vi "balance_controller.vi"(8 "Other variables":T1, 9 "systems":T6 {"SysD"."Transport Delay" format="%.2f"; "SysD"."D" format="%#.2g"; "SysD"."C" format="%#.2g"; "SysD"."B" format="%#.2g"; "SysD"."A" format="%#.2g"; "SysD"."properties"."Sampling Time" format="%#.6p"; "SysD"."properties"."Output Delays" format="%.4f"; "SysD"."properties"."Input Delays" format="%.4f"; "sysDo"."Transport Delay" format="%.2f"; "sysDo"."D" format="%#.2g"; "sysDo"."C" format="%#.2g"; "sysDo"."B" format="%#.2g"; "sysDo"."A" format="%#.2g"; "sysDo"."properties"."Sampling Time" format="%#.6p"; "sysDo"."properties"."Output Delays" format="%.4f"; "sysDo"."properties"."Input Delays" format="%.4f"; "sysDi"."Transport Delay" format="%.2f"; "sysDi"."D" format="%#.2g"; "sysDi"."C" format="%#.2g"; "sysDi"."B" format="%#.2g"; "sysDi"."A" format="%#.2g"; "sysDi"."properties"."Sampling Time" format="%#.6p"; "sysDi"."properties"."Output Delays" format="%.4f"; "sysDi"."properties"."Input Delays" format="%.4f"; "sysDC"."transfer function(s)"."delay" format="%.4f"; "sysDC"."transfer function(s)"."Denominator" format="%#_3g"; "sysDC"."transfer function(s)"."Numerator" format="%#_3g"; "sysDC"."properties"."Sampling Time" format="%#.6p"; "sysDC"."properties"."Output Delays" format="%.4f"; "sysDC"."properties"."Input Delays" format="%.4f"}) -> (3 "motor direction":dbl)   [LabVIEW 2016]
uses:
  <vilib>/addons/Control Design/_Model Construction/Model Typedefs.llb/CD State Space Model (MIMO).ctl
  <vilib>/addons/Control Design/_Model Construction/Model Typedefs.llb/CD General Elements.ctl
  <vilib>/addons/Control Design/_Model Construction/Model Typedefs.llb/CD Transfer Function Model (MIMO).ctl
  <vilib>/addons/Control Design/_Model Construction/Model Typedefs.llb/CD Transfer Function Model (SISO).ctl
  <vilib>/Analysis/Matrix/Datatypes/RealMatrix.ctl
  <vilib>/Simulation/DiscreteLinear/Implementation/NILVSim Discrete Transfer Function Direct.llb/SIM Discrete Transfer Function Diagram (SISO).vi
  <vilib>/Analysis/baseanly.llb/Real A x B.vi
  <vilib>/Simulation/ContinuousLinear/Implementation/Shared/SIM Transfer Function Support.llb/SIM TransferFunction Normalize to Buffer.vi
  <vilib>/Simulation/DiscreteLinear/Implementation/Shared/SIM Init Discrete States.vi
  <vilib>/Simulation/DiscreteLinear/Implementation/NILVSim Discrete Transfer Function Direct.llb/SIM Transfer Function Direct core (SISO).vi
  <vilib>/Simulation/ContinuousLinear/Implementation/Shared/SIM Transfer Function Support.llb/SIM TransferFunction Normalize.vi
  <vilib>/Simulation/Implementation/Shared/SIM Polynomials.llb/SIM Remove Zero Coefficients (DBL).vi
  <vilib>/Simulation/Implementation/Shared/SIM Polynomials.llb/SIM Divide Polynomials (DBL).vi
  <vilib>/Simulation/Implementation/Shared/SIM BuildSimErr.vi
  <vilib>/Analysis/Matrix/Numeric/Subtract/Subtract (Elementwise) - R,RM.vi
  <vilib>/Analysis/Matrix/Numeric/Add/Add - RM,RM.vi
  <vilib>/Simulation/Implementation/XNodeFramework/SimXNode/SimX.xnode
  <vilib>/Analysis/NI_AALBase.lvlib
  <vilib>/Simulation/ContinuousLinear/Implementation/NILVSim Integrator new.llb/SIM Integrator (vector).vi
  <vilib>/Analysis/baseanly.llb/A x Vector.vi
  <vilib>/Simulation/ContinuousLinear/Implementation/NILVSim Transfer Function.llb/SIM Transfer Function (SISO).vi
  <vilib>/Simulation/Nonlinear/Implementation/NILVSim Saturation.llb/SIM Saturation (scalar).vi
  <vilib>/Simulation/SignalDisplay/Implementation/NILVSim Time Waveform.llb/SIM Time Waveform (vector).vi
  <vilib>/Simulation/Nonlinear/Implementation/NILVSim Saturation.llb/SIM Saturation (vector).vi
  <vilib>/Analysis/baseanly.llb/Dot Product.vi
  <vilib>/Analysis/baseanly.llb/Real Dot Product.vi
  <vilib>/Simulation/Scripting/Companion Diagram/SimConfigNode/SimDog.xnode
  <vilib>/Simulation/Scripting/Companion Diagram/SimConfigNode/SimParams.ctl
  <vilib>/Simulation/Implementation/Shared/SIMSCR Execution Mode.ctl
  <vilib>/Simulation/Scripting/Companion Diagram/SimConfigNode/_simSolvers.ctl
  <vilib>/Simulation/Implementation/Shared/SIM Bundle Sim Info.vi
  <vilib>/Simulation/Implementation/Shared/SIM Unbundle Sim Info.vi
  <vilib>/Simulation/Implementation/Shared/NILVSim_FinalizeModel.vi
  <vilib>/Simulation/Implementation/Shared/NILVSim_GetModelError.vi
  <vilib>/Simulation/Implementation/Shared/NILVSim_Initialize.vi
  <vilib>/Simulation/Utility/Implementation/NILVSim Get Time and IsAcceptedStep.vi
  <vilib>/Simulation/Implementation/Shared/NILVSim_Manager.vi
  <vilib>/Simulation/Implementation/Shared/NI_SIM_Implementation.lvlib
  <vilib>/Simulation/Implementation/Shared/NILVSIM_BeginStep.vi
  <vilib>/Simulation/Param Hierarchy/Typedefs/SIMPH Param Control Actions.ctl
  <vilib>/Simulation/Implementation/Shared/NILVSim_ParamChanged.vi
  <vilib>/Utility/error.llb/Clear Errors.vi
  <vilib>/Simulation/Implementation/Shared/SIMSH Read Queue.vi
  <vilib>/Simulation/ContinuousLinear/Implementation/NILVSim Integrator new.llb/SIM Integrator Collector (vector).vi
  <vilib>/Simulation/ContinuousLinear/Implementation/NILVSim Integrator new.llb/SIM Integrator Distributor (vector).vi
  <vilib>/Simulation/Implementation/Shared/SIM limit type.ctl
  <vilib>/Simulation/ContinuousLinear/Implementation/NILVSim Transfer Function.llb/SIM Transfer Function Collector (SISO).vi
  <vilib>/Simulation/ContinuousLinear/Implementation/NILVSim Transfer Function.llb/SIM Transfer Function Distributor (SISO).vi
  <vilib>/Analysis/Matrix/NI_Matrix.lvlib
  <vilib>/Simulation/DiscreteLinear/Implementation/NILVSim Discrete Transfer Function Buffered.llb/SIM Discrete Transfer Function Buffered (SISO).vi
  <vilib>/Simulation/DiscreteLinear/Implementation/NILVSim Discrete Transfer Function Buffered.llb/SIM Discrete Transfer Function Distributor (SISO).vi
  <vilib>/addons/Control Design/_Model Construction/NI_LinSys_Model Typedefs.lvlib
panel:
  out "Waveform Chart 5":dbl[](graph)
  out "Waveform Chart 4":dbl[](graph)
  out "Waveform Chart 3":dbl[](graph)
  out "Waveform Chart 2":dbl[](graph)
  out "Waveform Chart":waveform(dbl)[](graph)
  in  "Whipple":T7
  out "Error":errorcluster
  out "output cluster":cluster{dbl[], dbl[]}
  in  "Inner Control Variable":T8
  in  "Outer Control Variable":T9
  in  "Other Variables":T10
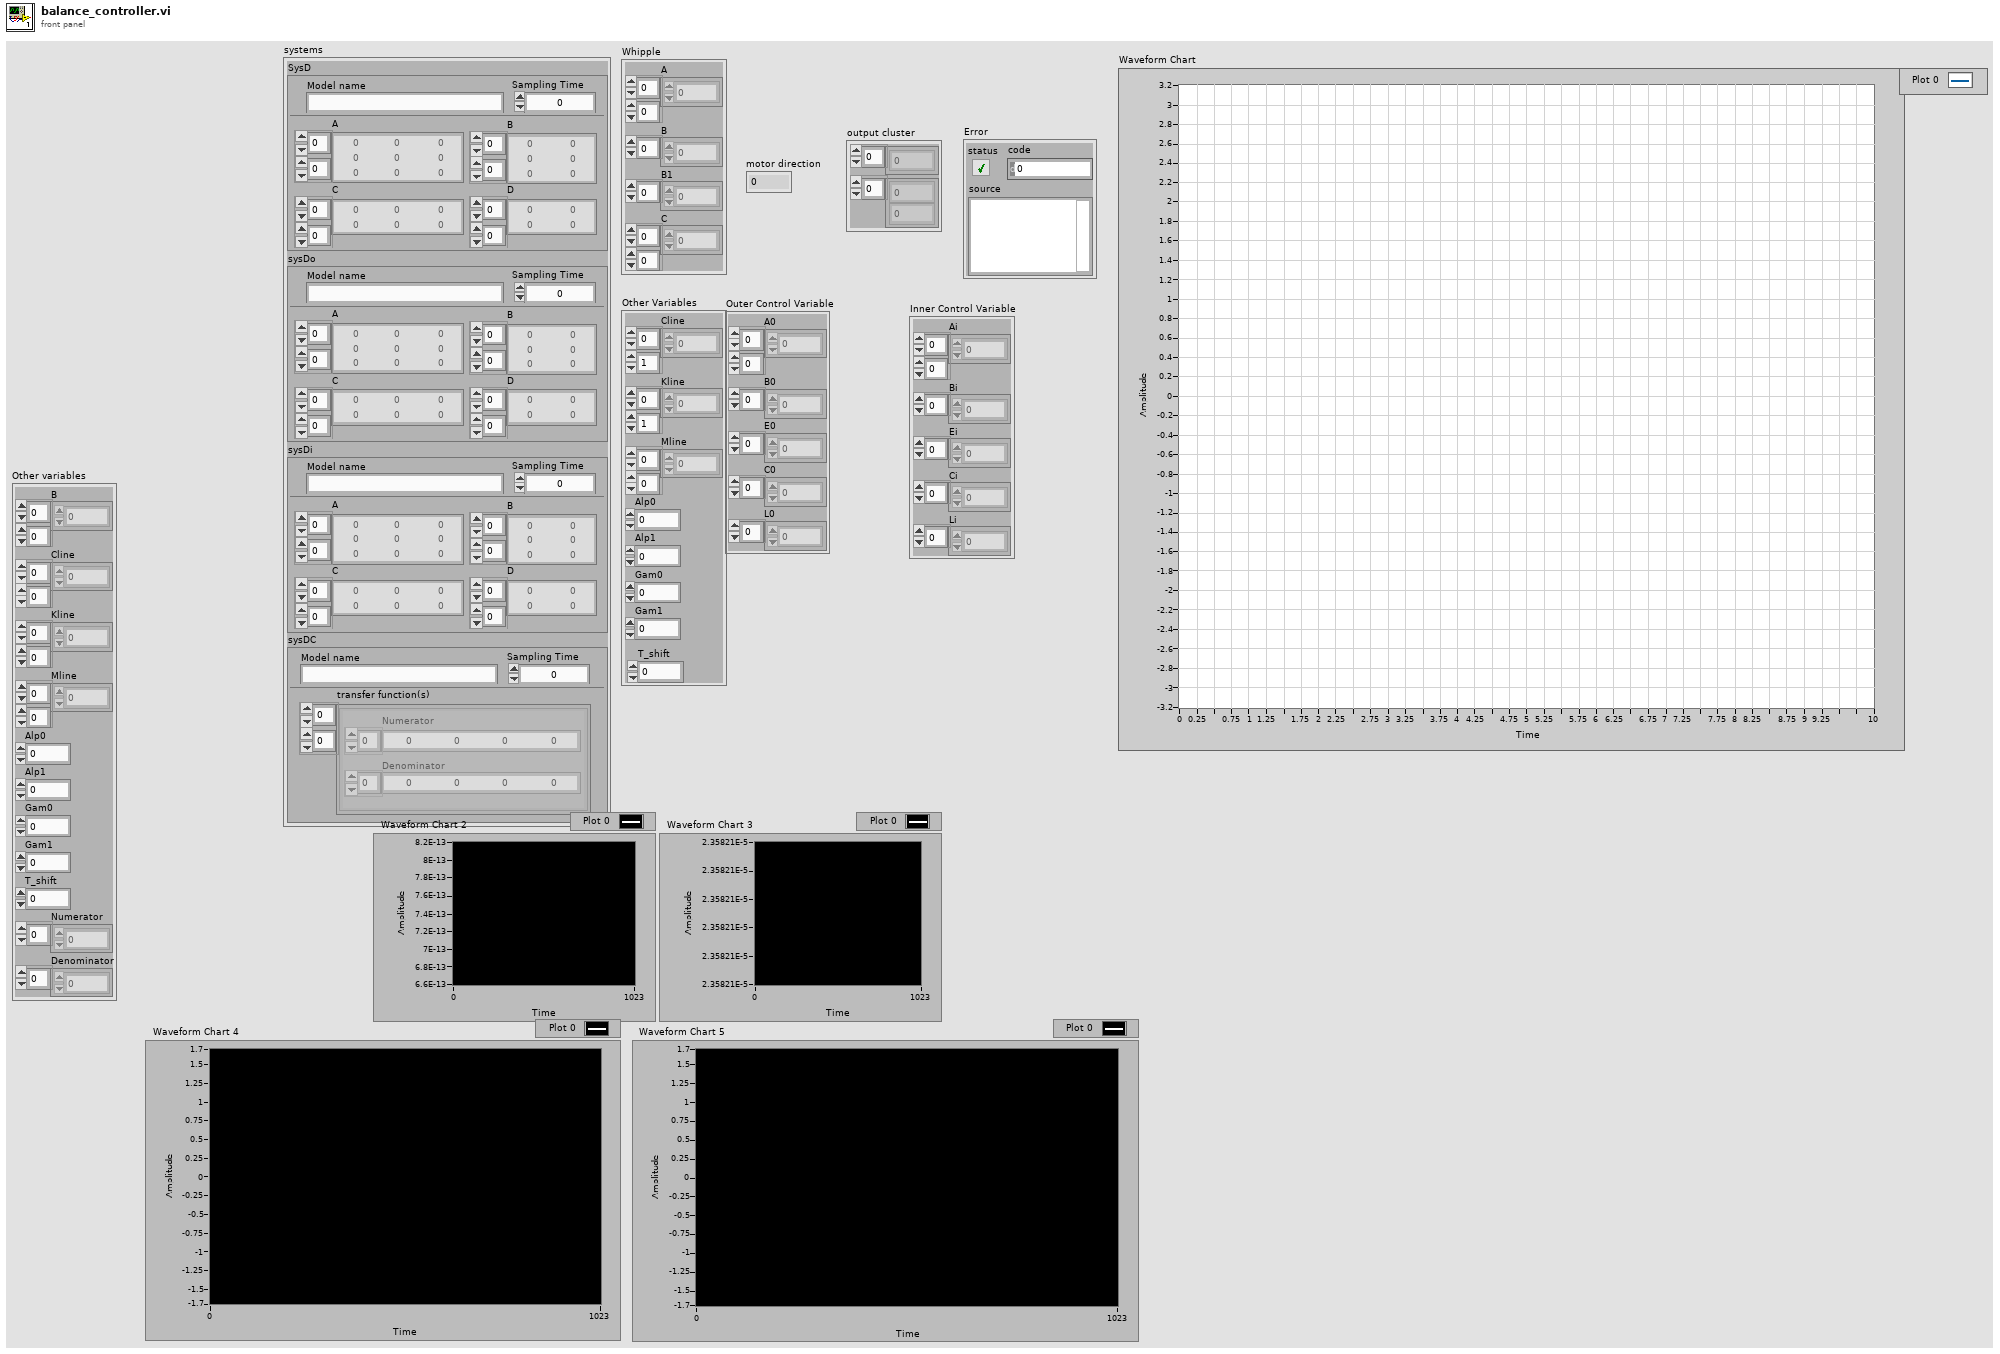
[diagram p1: front panel]
types:
  T1 = cluster{"B":dbl[][], "Cline":dbl[][], "Kline":dbl[][], "Mline":dbl[][], "Alp0":dbl, "Alp1":dbl, "Gam0":dbl, "Gam1":dbl, "T_shift":dbl, "Numerator":dbl[], "Denominator":dbl[]}
  T2 = typedef "NI_LinSys_Model Typedefs.lvlib/CD State Space Model (MIMO).ctl" = cluster{"properties":T3, "A":dbl[][], "B":dbl[][], "C":dbl[][], "D":dbl[][], "StateNames":string[], "Transport Delay":dbl[][]}
  T3 = typedef "NI_LinSys_Model Typedefs.lvlib/CD General Elements.ctl" = cluster{"Model name":string, "Input names":string[], "Output names":string[], "Input Delays":dbl[], "Output Delays":dbl[], "Sampling Time":dbl, "Notes":string}
  T4 = typedef "NI_LinSys_Model Typedefs.lvlib/CD Transfer Function Model (MIMO).ctl" = cluster{"properties":T3, "transfer function(s)":T5[][]}
  T5 = typedef "NI_LinSys_Model Typedefs.lvlib/CD Transfer Function Model (SISO).ctl" = cluster{"Numerator":dbl[], "Denominator":dbl[], "delay":dbl}
  T6 = cluster{"SysD":T2, "sysDo":T2, "sysDi":T2, "sysDC":T4}
  T7 = cluster{"A":dbl[][], "B":dbl[], "B1":dbl[], "C":i32[][]}
  T8 = cluster{"Ai":dbl[][], "Bi":dbl[], "Ei":i32[], "Ci":i32[], "Li":dbl[]}
  T9 = cluster{"A0":dbl[][], "B0":i32[], "E0":dbl[], "C0":i32[], "L0":dbl[]}
  T10 = cluster{"Cline":dbl[][], "Kline":dbl[][], "Mline":dbl[][], "Alp0":dbl, "Alp1":dbl, "Gam0":dbl, "Gam1":dbl, "T_shift":dbl}
  T11 = typedef "NI_Matrix.lvlib/RealMatrix.ctl" = dbl[][]
  T12 = cluster{"proportional gain (Kc)":dbl, "integral time (Ti, min)":dbl, "derivative time (Td, min)":dbl}
  T13 = typedef "SIMSCR Execution Mode.ctl" = enum16{"Simulate to Completion", "Single Time-Step Simulation (Fixed Step Only)"}
  T14 = typedef "SIMPH Param Control Actions.ctl" = enum16{"get params", "set params"}
  T15 = typedef "SIM limit type.ctl" = enum16{"upper", "lower", "both", "none"}
  T16 = typedef "SimParams.ctl" = cluster{"Initial Time (s)":dbl, "Final Time (s)":dbl, "Step Size (s)":dbl, "ODE Solver":T17, "Minimum Step Size (s)":dbl, "Maximum Step Size (s)":dbl, "Relative Tolerance":dbl, "Absolute Tolerance":dbl, "Software Timing":bool, "Initial Step Size (s)":dbl, "Automatic Fixed Step Size?":bool, "Automatic Discrete Step Size?":bool, "Discrete Step Size (s)":dbl, "Calculate using Time Step":bool, "Solver Wired?":bool, "Prev.Frm.Expected End":u64, "Prev.Frm.Actual End":u64, "Prev.Frm.Finished Late?":bool, "Prev.Iter.Expected End":u64, "Prev.Iter.Actual End":u64, "Prev.Iter.Finished Late?":bool, "Expected Iteration Start":u64, "Actual Iteration Start":u64, "Expected Frame Start":u64, "Actual Frame Start":u64, "Source Name":string, "Name":string, "Period":i64, "Deadline":i64, "Offset":i64, "Start":i64, "Priority":i32, "Timeout":i32, "Processor":i32, "Mode":enum32{"No Change", "Process missed periods, maintain original phase", "Discard missed periods, maintain original phase", "Process missed periods, ignore original phase", "Discard missed periods, ignore original phase"}, "Wakeup reason":enum32{"Normal", "Aborted", "Asynchronous wakeup", "Timing source error", "Timed loop error", "Timeout"}, "Error":errorcluster, "Source Type":string, "Secondary Source Type":string, "Global End Time":u64, "Global Start Time":u64, "Full Solver Reset":bool, "Execution Mode":T13, "Nan/Inf Check":bool, "Custom Solver Library":string, "Solver Is Variable":bool, "custom solver name":string, "Signal Collection Decimation":u32}
  T17 = typedef "_simSolvers.ctl" = enum16{"Runge-Kutta 1 (Euler)", "Runge-Kutta 2", "Runge-Kutta 3", "Runge-Kutta 4", "Runge-Kutta 23 (variable)", "Runge-Kutta 45 (variable)", "BDF (variable)", "Adams-Moulton (variable)", "Rosenbrock (variable)", "Discrete States Only", "SDIRK 4 (variable)", "Radau 5 (variable)", "Radau 9 (variable)", "Radau 13 (variable)", "Radau [Variable Order] (variable)", "Gear's Method (variable)", "Linearizer", "State Query", "Trim Eval", "Custom Solver"}
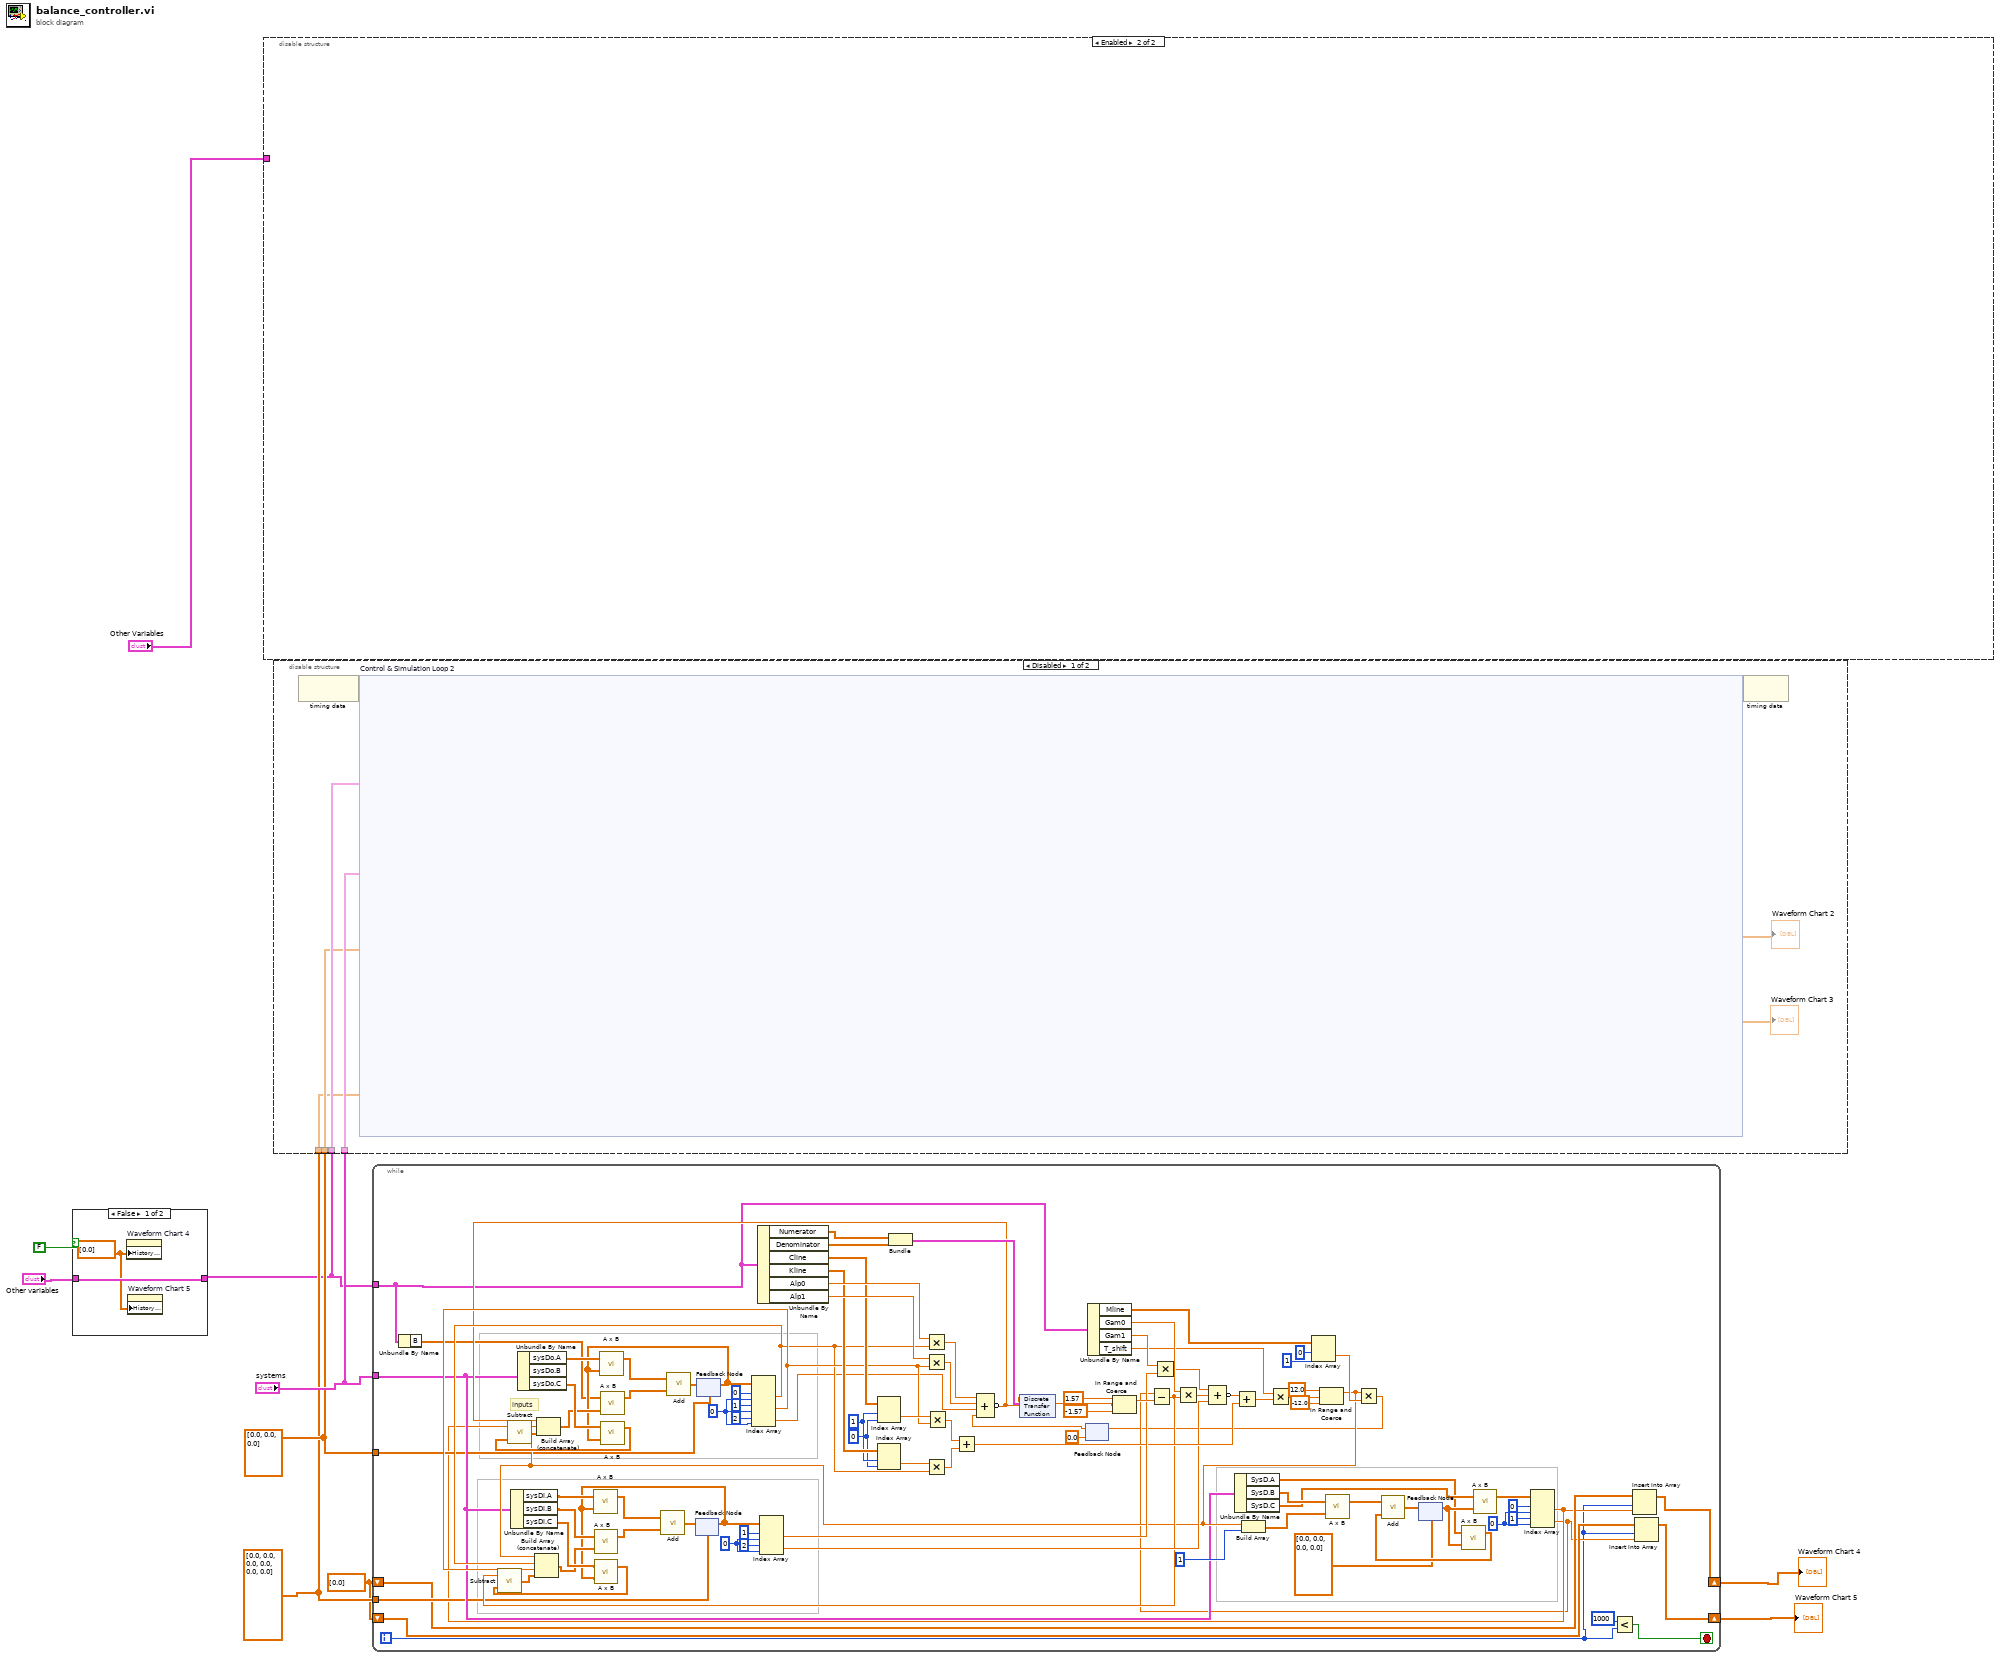
[diagram p0: block diagram]
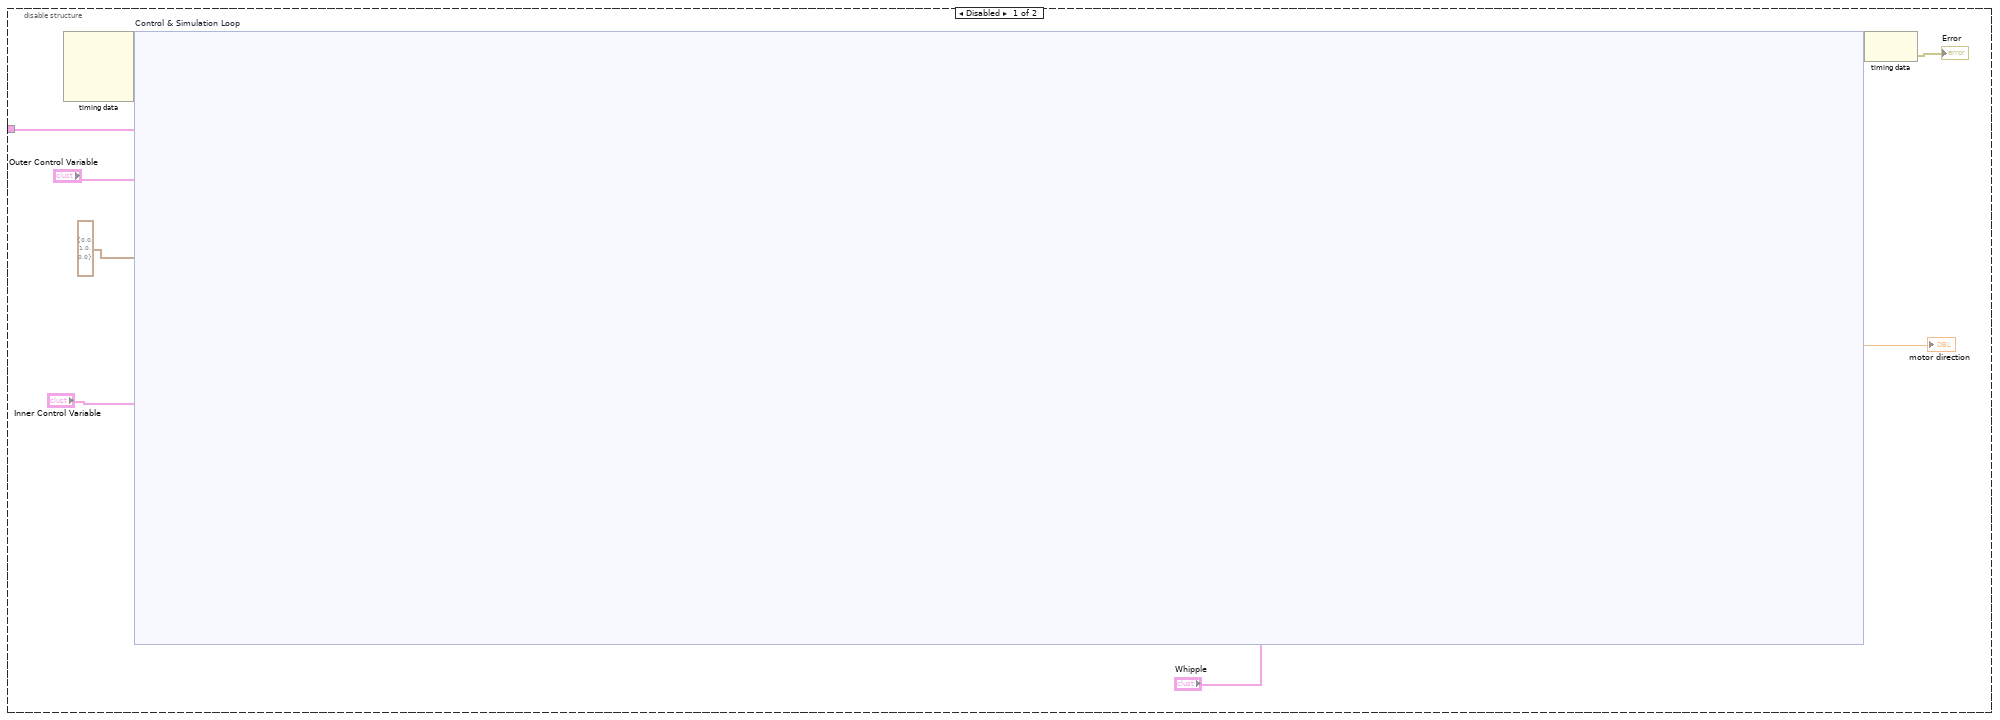
[diagram p4: hidden frame]
diagram:
  w6 = dbl[] [0.0]
  w8 = T11 [[0.0], [0.0], [0.0]] ("A + B")
  w7 = T11 [[0.0], [0.0], [0.0], [0.0], [0.0], [0.0]] ("A + B")
  n1 = case shown="False" FALSE {
    tunnel: [w12 w13] -> w2
    tunnel: "Other variables" -> [w12 w13]
    frame False {
      w11 = dbl[] [0.0] ("History Data")
      n2 = property on="Waveform Chart 4" class="WFChart (strict)"("History Data"=w11) -> ()  [unwired: 2 in, 2 out]
      n3 = property on="Waveform Chart 5" class="WFChart (strict)"("History Data"=w11) -> ()  [unwired: 2 in, 2 out]
    }
    frame True {
    }
  }
  n4 = disable-structure shown="Enabled" {
    disable-tunnel: "Other Variables" -> [w20 _]
    frame Disabled {
      n5 = node-c288() -> (w22:variant)  [unwired: 4 in]
      n6 = node-c254 "Control & Simulation Loop"(w22, w20, "Inner Control Variable", "Outer Control Variable", "Whipple", T12 {"proportional gain (Kc)"=0.0, "integral time (Ti, min)"=1.0, "derivative time (Td, min)"=0.0} ("PID gains")) -> (w21:variant, →"motor direction":dbl)
      n7 = node-c288(w21) -> (→"Error":errorcluster)
    }
    frame Enabled {
    }
  }
  n8 = disable-structure shown="Disabled" {
    disable-tunnel: "systems" -> [w784 _]
    disable-tunnel: w2 -> [w783 _]
    disable-tunnel: w8 -> [w782 _]
    disable-tunnel: w7 -> [w781 _]
    frame Disabled {
      n9 = node-c288() -> (w788:variant)  [unwired: 1 in]
      n10 = node-c254 "Control & Simulation Loop 2"(w788, w784, w783, w781, w782) -> (w787:variant, →"Waveform Chart 2":dbl[], →"Waveform Chart 3":dbl[])
      n11 = node-c288(w787) -> ()  [unwired: 1 out]
    }
    frame Enabled {
    }
  }
  n12 = while {
    tunnel: "systems" -> [w1357]
    tunnel: w2 -> [w1345]
    tunnel: w8 -> [w1356]
    tunnel: w7 -> [w1355]
    shift-right: [w1346] -> w4
    shift-left: w6 -> [w1349]
    shift-right: [w1350] -> w5
    shift-left: w6 -> [w1352]
    i -> [w1347]
    stop <- w1354 stop-if-true
    w1367 = 0 ("index (row) 11")
    w1405 = 0 ("index (row) 9")
    w1406 = 1 ("index (row) 8")
    w1415 = 0 ("index (row) 5")
    w1420 = 0 ("index (row)")
    # "inputs"
    n13 = Unbundle By Name(w1345) -> ("B"=w1344:dbl[][])
    n14 = Unbundle By Name ("Unbundle By Name 2")(w1357) -> ("sysDi.A"=w1429:dbl[][], "sysDi.B"=w1428:dbl[][], "sysDi.C"=w1427:dbl[][])
    n15 = Unbundle By Name(w1357) -> ("sysDo.A"=w1438:dbl[][], "sysDo.C"=w1434:dbl[][])  [unwired: 1 out]
    n16 = feedback #1 ("Feedback Node 2")(w1355) -> (w1416:T11)
    n17 = call-poly <vilib>:"A x B.vi"("B"=w1416, "A"=w1429) -> ("A x B"=w1431:T11)  [unwired: 1 out]
    n18 = call-poly <vilib>:"A x B.vi"("B"=w1416, "A"=w1427) -> ("A x B"=w1426:T11)  [unwired: 1 out]
    n19 = feedback #2(w1356) -> (w1421:T11)
    n20 = call-poly <vilib>:"A x B.vi"("B"=w1421, "A"=w1438) -> ("A x B"=w1436:T11)  [unwired: 1 out]
    n21 = call-poly <vilib>:"A x B.vi"("B"=w1421, "A"=w1434) -> ("A x B"=w1433:T11)  [unwired: 1 out]
    n22 = Index Array ("Get Matrix Elements")(array=w1421, index (row) #1=0 ("index (row) 2"), index (col) #1=w1420, index (row) #2=1 ("index (row) 3"), index (col) #2=w1420, index (row) #3=2 ("index (row) 4"), index (col) #3=w1420) -> (element #1=w1401:dbl, element #2=w1402:dbl, element #3=w1398:dbl)
    n23 = Unbundle By Name ("Unbundle By Name 3")(w1345) -> ("Numerator"=w1361:dbl[], "Denominator"=w1360:dbl[], "Cline"=w1408:dbl[][], "Kline"=w1407:dbl[][], "Alp0"=w1411:dbl, "Alp1"=w1412:dbl)
    n24 = Index Array ("Get Matrix Elements 2")(array=w1416, index (row) #1=1 ("index (row) 6"), index (col) #1=w1415, index (row) #2=2 ("index (row) 7"), index (col) #2=w1415) -> (element #1=w1390:dbl, element #2=w1382:dbl)
    n25 = Index Array ("Get Matrix Elements 3")(array=w1408, index (row)=w1406, index (col)=w1405) -> (element=w1403:dbl)
    n26 = Index Array ("Get Matrix Elements 4")(array=w1407, index (row)=w1406, index (col)=w1405) -> (element=w1404:dbl)
    n27 = Bundle("Numerator"=w1361, "Denominator"=w1360) -> (w1359:cluster{"Numerator":dbl[], "Denominator":dbl[]})  [unwired: 1 in]
    n28 = Multiply ("Multiply 4")(x=w1411, y=w1401) -> (x*y=w1410:dbl)
    n29 = Multiply ("Multiply 5")(x=w1412, y=w1402) -> (x*y=w1409:dbl)
    n30 = Multiply ("Multiply 7")(x=w1404, y=w1401) -> (x*y=w1399:dbl)
    n31 = Multiply ("Multiply 6")(x=w1403, y=w1402) -> (x*y=w1400:dbl)
    n32 = Add ("Add.vi 3")(x=w1400, y=w1399) -> (x+y=w1388:dbl)
    n33 = feedback #3(0.0 ("output y(k)")) -> (w1341:dbl)
    n34 = Compound Arithmetic op=ADD(w1410, w1409, w1398, w1341) -> (invert w1358:dbl)
    n35 = xnode ("Discrete Transfer Function")("input u(k)"=w1358, "Transfer Function"=w1359) -> ("output y(k)"=w1340:dbl)  [unwired: 2 in, 1 out]
    n36 = Unbundle By Name ("Unbundle By Name 5")(w1345) -> ("Mline"=w1362:dbl[][], "Gam0"=w1394:dbl, "Gam1"=w1391:dbl, "T_shift"=w1386:dbl)
    n37 = In Range and Coerce(upper limit=1.57, x=w1340, lower limit=-1.57 ("upper limit 2")) -> (coerced(x)=w1395:dbl)  [unwired: 1 out]
    n38 = Multiply ("Multiply 9")(x=w1391, y=w1390) -> (x*y=w1383:dbl)
    n39 = Unbundle By Name ("Unbundle By Name 6")(w1357) -> ("SysD.A"=w1370:dbl[][], "SysD.B"=w1377:dbl[][], "SysD.C"=w1371:dbl[][])
    n40 = Index Array ("Get Matrix Elements 5")(array=w1362, index (row)=0, index (col)=1 ("index (row) 10")) -> (element=w1379:dbl)
    n41 = feedback #4 ("Feedback Node 3")(T11 [[0.0], [0.0], [0.0], [0.0]] ("A + B")) -> (w1372:T11)
    n42 = call-poly <vilib>:"A x B.vi"("B"=w1372, "A"=w1370) -> ("A x B"=w1373:T11)  [unwired: 1 out]
    n43 = call-poly <vilib>:"A x B.vi"("B"=w1372, "A"=w1371) -> ("A x B"=w1366:T11)  [unwired: 1 out]
    n44 = Index Array ("Get Matrix Elements 6")(array=w1366, index (row) #1=0 ("index (row) 12"), index (col) #1=w1367, index (row) #2=1 ("index (row) 13"), index (col) #2=w1367) -> (element #1=w1351:dbl, element #2=w1348:dbl)
    n45 = call-poly <vilib>:"Subtract.vi"("Real Matrix A"=w1433, "Real Scalar c"=w1351) -> ("c - A"=w1423:T11)
    n46 = Subtract(x=w1348, y=w1395) -> (x-y=w1365:dbl)
    n47 = call-poly <vilib>:"Subtract.vi"("Real Matrix A"=w1426, "Real Scalar c"=w1365) -> ("c - A"=w1424:T11)
    n48 = Multiply ("Multiply 8")(x=w1394, y=w1365) -> (x*y=w1384:dbl)
    n49 = Compound Arithmetic op=ADD ("Compound Arithmetic 2")(w1383, w1384, w1382) -> (invert w1389:dbl)
    n50 = Add ("Add.vi 4")(x=w1389, y=w1388) -> (x+y=w1387:dbl)
    n51 = Multiply ("Multiply 10")(x=w1386, y=w1387) -> (x*y=w1385:dbl)
    n52 = In Range and Coerce ("In Range and Coerce 2")(upper limit=12.0 ("upper limit 3"), x=w1385, lower limit=-12.0 ("upper limit 4")) -> (coerced(x)=w1364:dbl)  [unwired: 1 out]
    n53 = Build Array (concatenate) ("Build Matrix")(w1364, w1401, w1402, w1424) -> (w1425:T11)
    n54 = Build Array (concatenate) ("Build Matrix 2")(w1358, w1364, w1423) -> (w1422:T11)
    n55 = call-poly <vilib>:"A x B.vi"("B"=w1425, "A"=w1428) -> ("A x B"=w1432:T11)  [unwired: 1 out]
    n56 = call-poly <vilib>:"A x B.vi"("B"=w1422, "A"=w1344) -> ("A x B"=w1437:T11)  [unwired: 1 out]
    n57 = call-poly <vilib>:"Add.vi"("Real Matrix B"=w1432, "Real Matrix A"=w1431) -> ("A + B"=w1430:T11)
    n58 = call-poly <vilib>:"Add.vi"("Real Matrix B"=w1437, "Real Matrix A"=w1436) -> ("A + B"=w1435:T11)
    n59 = feedback-in #1 ("3")(w1430) -> ()
    n60 = feedback-in #2 ("2")(w1435) -> ()
    n61 = Build Array ("Build Matrix 3")(w1364, 1 ("Real Matrix Element")) -> (w1376:T11)
    n62 = call-poly <vilib>:"A x B.vi"("B"=w1376, "A"=w1377) -> ("A x B"=w1375:T11)  [unwired: 1 out]
    n63 = Multiply ("Multiply 11")(x=w1364, y=w1379) -> (x*y=w1342:dbl)
    n64 = feedback-in #3(w1342) -> ()
    n65 = call-poly <vilib>:"Add.vi"("Real Matrix B"=w1373, "Real Matrix A"=w1375) -> ("A + B"=w1374:T11)
    n66 = feedback-in #4 ("4")(w1374) -> ()
    n67 = Less?(x=1000, y=w1347) -> (x < y?=w1354:bool)
    n68 = Insert Into Array(array=w1352, index=w1347, new element=w1351) -> (w1350:dbl[])
    n69 = Insert Into Array(array=w1349, index=w1347, new element=w1348) -> (w1346:dbl[])
  }
  "Waveform Chart 4" <- w5
  "Waveform Chart 5" <- w4
